vi "Get Direction.vi"(11 "Direction":T1) -> (3 "Direction":cluster{"Numeric":i32, "Numeric":i32})   [LabVIEW 2024]
uses:
  ENUM_Direction.ctl
  <vilib>/Utility/error.llb/Trim Whitespace One-Sided.vi
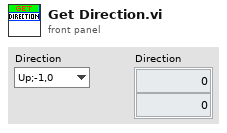
[diagram p1: front panel]
types:
  T1 = typedef "ENUM_Direction.ctl" = enum16{"Up;-1,0", "Right;0,1", "Down;1,0", "Left;0,-1"}
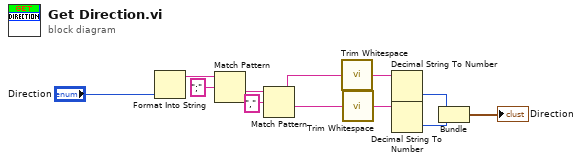
[diagram p0: block diagram]
diagram:
  n1 = Format Into String("Direction") -> (resulting string=w10:string)  [unwired: 3 in, 1 out]
  n2 = Match Pattern(string=w10, regular expression=";") -> (after substring=w2:string)  [unwired: 1 in, 3 out]
  n3 = Match Pattern(string=w2, regular expression=",") -> (before substring=w3:string, after substring=w1:string)  [unwired: 1 in, 2 out]
  n4 = call <vilib>:"Trim Whitespace.vi"("string"=w3) -> ("trimmed string"=w8:string)  [unwired: 1 in]
  n5 = call <vilib>:"Trim Whitespace.vi"("string"=w1) -> ("trimmed string"=w7:string)  [unwired: 1 in]
  n6 = Decimal String To Number(string=w8) -> (number=w6:i32)  [unwired: 2 in, 1 out]
  n7 = Decimal String To Number(string=w7) -> (number=w5:i32)  [unwired: 2 in, 1 out]
  n8 = Bundle(w6, w5) -> (→"Direction":cluster{i32, i32})  [unwired: 1 in]
